vi "Build SubNode Array.vi"(9 "Names Array In":string[](array[string]), 10 "Parent NodeID In":string) -> (2 "SubNode Array Out":string[](array[string]))   [LabVIEW 2024]
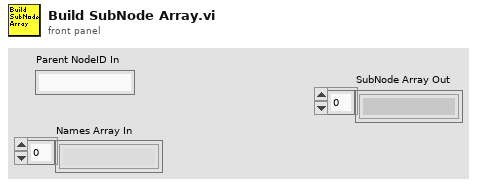
[diagram p1: front panel]
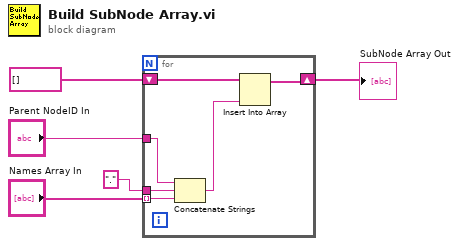
[diagram p0: block diagram]
diagram:
  n1 = for {
    tunnel: "Names Array In" -> [w11] mode=indexing
    tunnel: "." -> [w10]
    tunnel: "Parent NodeID In" -> [w9]
    shift-right: [w7] -> w1
    shift-left: string[] [] -> [w8]
    n2 = Concatenate Strings(w9, w10, w11) -> (w6:string)
    n3 = Insert Into Array(array=w8, new element=w6) -> (w7:string[])  [unwired: 1 in]
  }
  "SubNode Array Out" <- w1
